vi "Load Class.vi"(8 "error in (no error)":errorcluster, 11 "Configuration in":refnum<class "Configuration.lvclass">) -> (0 "error out":errorcluster, 2 "Loaded Class":refnum<class>, 3 "Configuration out":refnum<class "Configuration.lvclass">)   [LabVIEW 2019, in "Configuration.lvlib" / "Configuration.lvclass"]
doc: "Use config.ini file data to identify child class component. \nReturn child class component."
uses:
  Configuration.lvclass
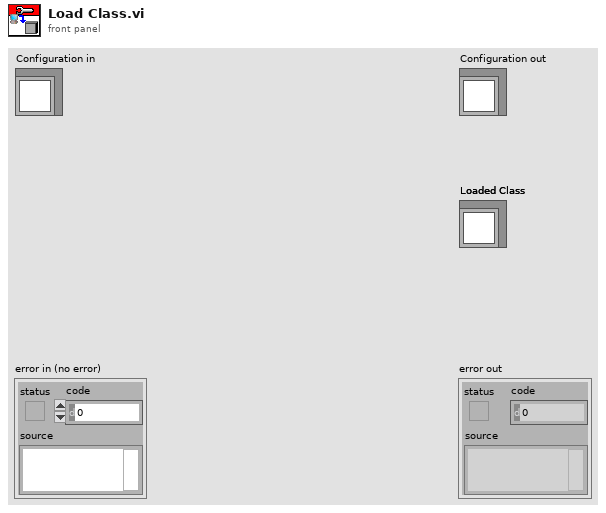
[diagram p1: front panel]
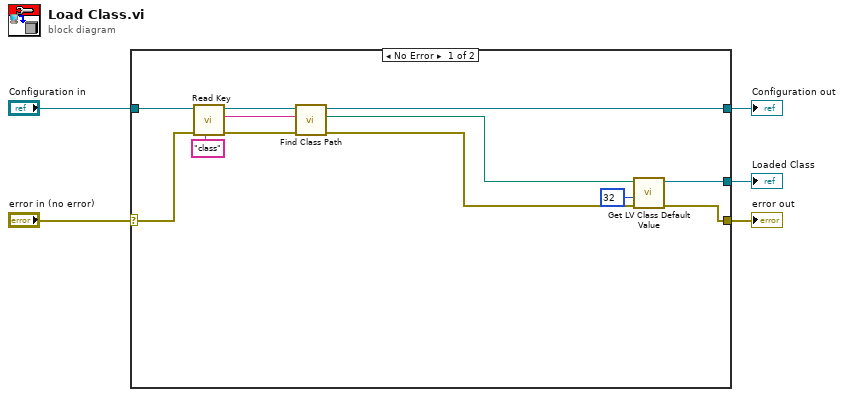
[diagram p0: block diagram]
diagram:
  n1 = case shown="No Error" "error in (no error)" {
    selector: "error in (no error)" -> [w13 w19]
    tunnel: [w16 w19] -> w4
    tunnel: [w8 w18] -> w2
    tunnel: "Configuration in" -> [w14 w18]
    tunnel: [w17 _] -> w1
    frame No Error {
      n2 = call "Read Key.vi"("Key Name"="class", "error in (no error)"=w13, "Configuration in"=w14) -> ("error out"=w10:errorcluster, "Key Value"=w7:string, "Configuration out"=w11:refnum<class "Configuration.lvclass">)  [unwired: 6 in]
      n3 = call "Find Class Path.vi"("error in"=w10, "Class Name"=w7, "Configuration in"=w11) -> ("error out"=w9:errorcluster, "Class Path"=w6:path, "Configuration out"=w8:refnum<class "Configuration.lvclass">)  [unwired: 6 in]
      n4 = call <vilib>:"Get LV Class Default Value.vi"("error in (no error)"=w9, "options"=u32 32, "class path"=w6) -> ("error out"=w16:errorcluster, "object"=w17:refnum<class>)  [unwired: 7 in]
    }
    frame Error {
    }
  }
  "error out" <- w4
  "Configuration out" <- w2
  "Loaded Class" <- w1
